vi "AndorResizeImage.vi"(8 "error in (no error)":errorcluster, 9 "Image Area Width":u32, 10 "Image Area Height":u32, 11 "Refnum in":T1) -> (0 "error out":errorcluster, 3 "Refnum out":T1)   [LabVIEW 2018, in "AndorOWN.lvlib"]
uses:
  AndorOWN.lvlib
  <vilib>/vision/Image Controls.llb/IMAQ Image.ctl
  <vilib>/vision/NI_Vision_Development_Module.lvlib
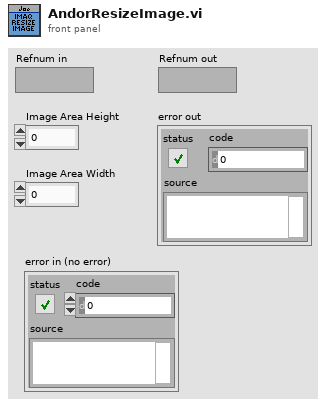
[diagram p1: front panel]
types:
  T1 = typedef "IMAQ Image.ctl" = refnum<image>
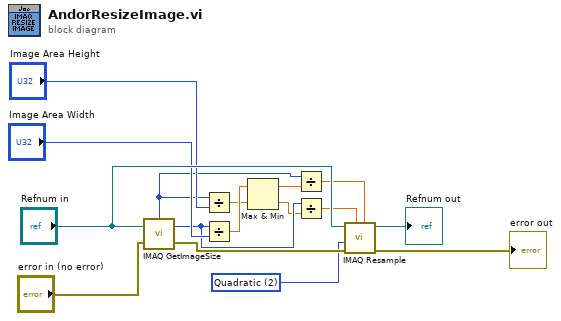
[diagram p0: block diagram]
diagram:
  w1 = u32 2 items=["Zero Order", "Bi-Linear", "Quadratic", "Cubic Spline"] ("Interpolation Type")
  n1 = call "IMAQ GetImageSize"("Image"="Refnum in", "error in (no error)"="error in (no error)") -> ("Y Resolution"=w10:i32, "X Resolution"=w7:i32, "error out"=w11:errorcluster)  [unwired: 2 in]
  n2 = Divide(x=w7, y="Image Area Height") -> (x/y=w3:dbl)
  n3 = Divide(x=w10, y="Image Area Width") -> (x/y=w4:dbl)
  n4 = Max & Min(x=w4, y=w3) -> (max(x,y)=w5:dbl, min(x,y)=w9:dbl)
  n5 = Divide(x=w7, y=w5) -> (x/y=w6:dbl)
  n6 = Divide(x=w10, y=w9) -> (x/y=w8:dbl)
  n7 = call "IMAQ Resample"("X Resolution"=w6, "Y Resolution"=w8, "error in (no error)"=w11, "Interpolation Type"=w1, "Image Src"="Refnum in") -> ("error out"=→"error out":errorcluster, "Image Dst Out"=→"Refnum out":T1)  [unwired: 5 in]
